vi "Queue and Case Management.vi"(8 "States input":T1=enum."Startup", 11 "Queue element":u8) -> (0 "States output":T1=enum."Startup", 3 "Slider output":u8)   [LabVIEW 2021]
doc: "This VI receives the queue element, manages the data, and transfers it to the main state machine and the car position slider."
uses:
  Controls/Enum State Machine.ctl
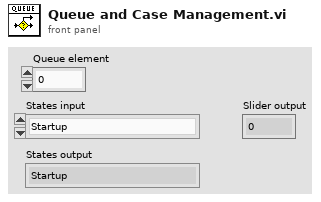
[diagram p1: front panel]
types:
  T1 = typedef "Enum State Machine.ctl" = enum16{"Entry", "Under Body Wash", "Bug Remover", "Pre-Soak", "High Pressure Wash", "Low Pressure Wax", "Spot Free Rinse", "Tire Shine Foam", "Air Dry", "Exit", "Startup", "Wait for Start", "Stop"}
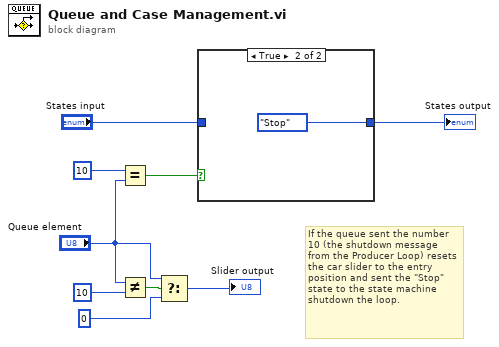
[diagram p0: block diagram]
diagram:
  # "If the queue sent the number 10 (the shutdown message from the Producer Loop) resets the car slider to the entry position and sent the \"Stop\" state to the state machine shutdown the loop."
  n1 = Equal?(x=u8 10, y="Queue element") -> (x = y?=w3:bool)
  n2 = Not Equal?(x="Queue element", y=u8 10) -> (x != y?=w6:bool)
  n3 = Select(t="Queue element", s=w6, f=u8 0) -> (s? t:f=→"Slider output":u8)
  n4 = case shown="True" w3 {
    tunnel: "States input" -> [w10 _]
    tunnel: [w10 Enum_State_Machine."Stop" ("States input")] -> w1
    frame False {
    }
    frame True {
    }
  }
  "States output" <- w1
